vi "Save As EDF.vi"(8 "error in (no error)":errorcluster, 10 "iMode":i32, 11 "szPath":string) -> (0 "error out":errorcluster, 2 "function return":u32, 3 "szPath out":string)   [LabVIEW 2018, in "AndorSDK.lvlib"]
doc: "EXPNETTYPE unsigned int WINAPI SaveAsEDF(char * szPath, int iMode);"
uses:
  AndorSDK.lvlib
  ATMCD32D.dll
  OwnVIs/AndorOWN.lvlib
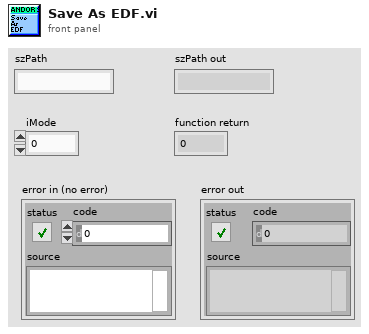
[diagram p1: front panel]
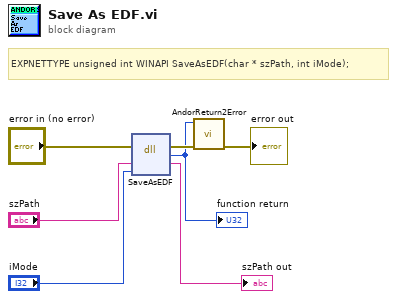
[diagram p0: block diagram]
diagram:
  # "EXPNETTYPE unsigned int WINAPI SaveAsEDF(char * szPath, int iMode);"
  n1 = dll-call lib="C:/Users/johan/Downloads/LabVIEW software/LabVIEW software/IX-81 Software/lib/ANDOR/Andor SDK/ATMCD32D.*" fn="SaveAsEDF"(error in="error in (no error)", "szPath"="szPath", "iMode"="iMode") -> (error out=w4:errorcluster, w3:u32, "szPath"=→"szPath out":string)  [unwired: 3 in, 1 out]
  "function return" <- w3
  n2 = call "AndorReturn2Error.vi"("error in (no error)"=w4, "Camera return"=w3) -> ("error out"=→"error out":errorcluster)  [unwired: 9 in]
